vi "Write Cam Attr IF.lvclass.vi"(8 "error in (no error)":errorcluster, 10 "Cam Attr IF.lvclass":refnum<class "Cam Attr IF.lvclass">, 11 "Camera Settings Dialog in":refnum<class "Camera Settings Dialog.lvclass">) -> (0 "error out":errorcluster, 3 "Camera Settings Dialog out":refnum<class "Camera Settings Dialog.lvclass">)   [LabVIEW 2020, in "Camera Settings Dialog UI.lvlib" / "Camera Settings Dialog.lvclass"]
uses:
  Camera Settings Dialog.lvclass
  Camera Settings Dialog.lvclass/Camera Settings Dialog.ctl
  Camera Attr IF/Cam Attr IF.lvclass
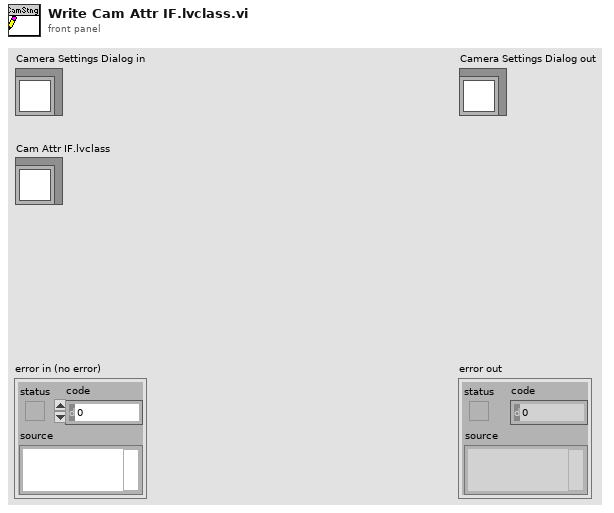
[diagram p1: front panel]
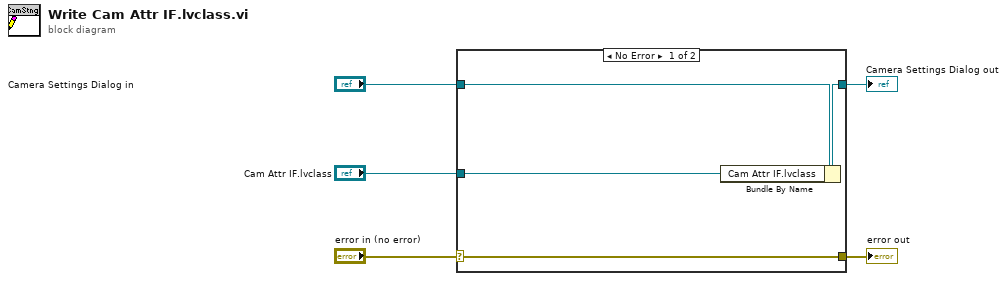
[diagram p0: block diagram]
diagram:
  n1 = case shown="No Error" "error in (no error)" {
    selector: "error in (no error)" -> [w9 w10]
    tunnel: [w9 w10] -> w4
    tunnel: [w7 w11] -> w2
    tunnel: "Camera Settings Dialog in" -> [w8 w11]
    tunnel: "Cam Attr IF.lvclass" -> [w6 _]
    frame No Error {
      n2 = Bundle By Name(cluster=w8, "Cam Attr IF.lvclass"=w6) -> (w7:refnum<class "Camera Settings Dialog.lvclass">)
    }
    frame Error {
    }
  }
  "error out" <- w4
  "Camera Settings Dialog out" <- w2
